vi "Translate Tile.vi"(0 "Tile in":T2 items=["Empty", "Portal", "Open", "Wall", ">", "<", ">-^", ">-v", "^-<", "v-<"], 1 "Direction in":T1) -> (2 "Direction out":T1, 3 "Tile out":T2 items=["Empty", "Portal", "Open", "Wall", ">", "<", ">-^", ">-v", "^-<", "v-<"])   [LabVIEW 2020, in "AoC 2022.lvlib"]
uses:
  AoC 2022.lvlib
  Map Tile.ctl
  Map Direction.ctl
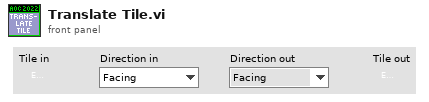
[diagram p1: front panel]
types:
  T1 = typedef "AoC 2022.lvlib/Map Direction.ctl" = enum16{"Facing", "Right", "Left", "Up", "Down"}
  T2 = typedef "AoC 2022.lvlib/Map Tile.ctl" = u16
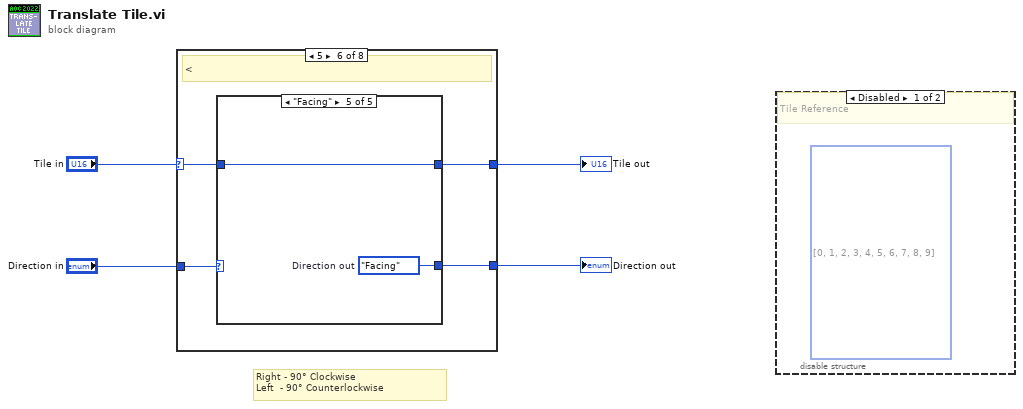
[diagram p0: block diagram]
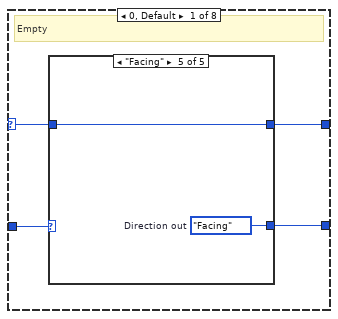
[diagram p2: hidden frame]
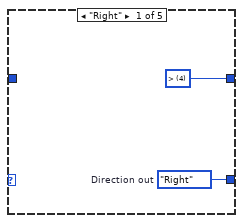
[diagram p3: hidden frame]
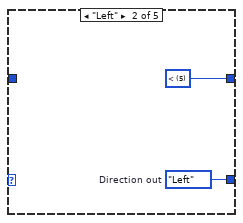
[diagram p4: hidden frame]
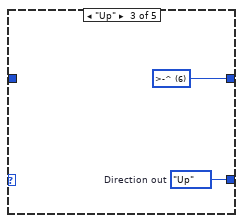
[diagram p5: hidden frame]
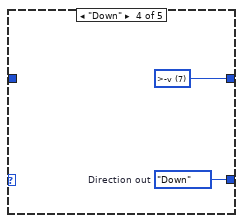
[diagram p6: hidden frame]
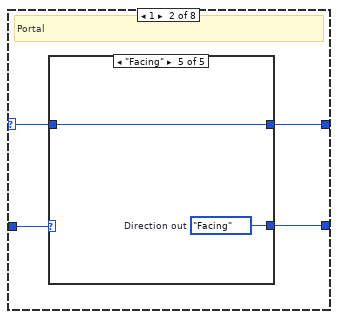
[diagram p7: hidden frame]
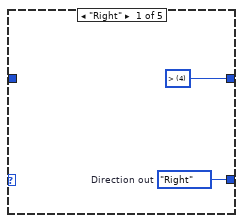
[diagram p8: hidden frame]
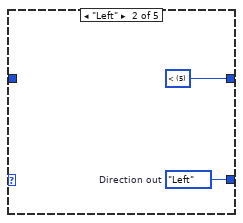
[diagram p9: hidden frame]
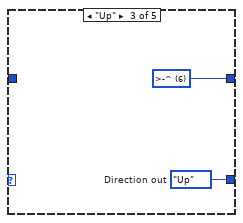
[diagram p10: hidden frame]
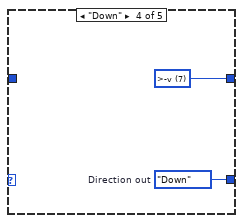
[diagram p11: hidden frame]
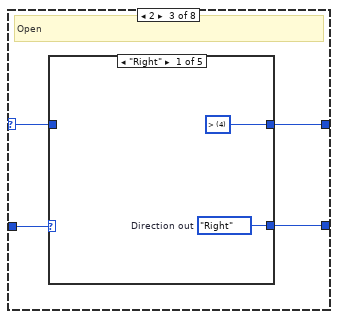
[diagram p12: hidden frame]
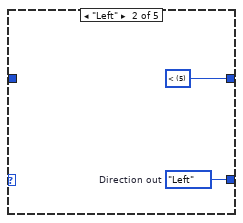
[diagram p13: hidden frame]
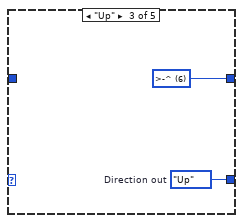
[diagram p14: hidden frame]
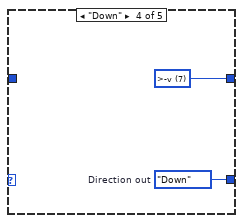
[diagram p15: hidden frame]
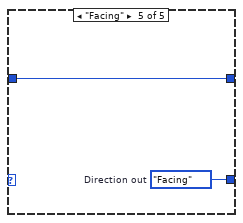
[diagram p16: hidden frame]
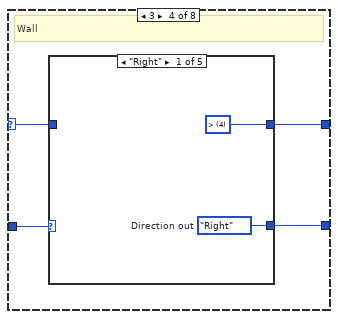
[diagram p17: hidden frame]
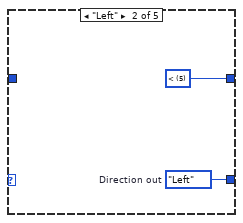
[diagram p18: hidden frame]
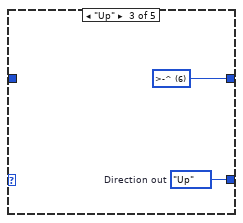
[diagram p19: hidden frame]
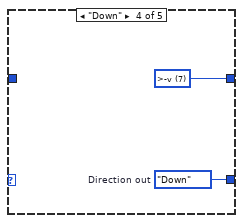
[diagram p20: hidden frame]
diagram:
  # "Right - 90° Clockwise\nLeft  - 90° Counterlockwise"
  n1 = case shown="5" "Tile in" {
    selector: "Tile in" -> [w5 w19 w33 w47 w61 w75 w89 w103]
    tunnel: [w8 w22 w36 w50 w64 w78 w92 w106] -> w3
    tunnel: "Direction in" -> [w7 w21 w35 w49 w63 w77 w91 w105]
    tunnel: [w6 w20 w34 w48 w62 w76 w90 w104] -> w1
    frame 0, Default {
      # "Empty"
      n2 = case shown="\"Facing\"" w7 {
        tunnel: [w10 w12 w14 w16 w17] -> w8
        tunnel: [w9 w11 w13 w15 w18] -> w6
        tunnel: w5 -> [_ _ _ _ w17]
        frame "Right" {
          w9 = Map_Direction."Right"  # Direction out
          w10 = T2 4 items=["Empty", "Portal", "Open", "Wall", ">", "<", ">-^", ">-v", "^-<", "v-<"] ("Tile")
        }
        frame "Left" {
          w11 = Map_Direction."Left"  # Direction out
          w12 = T2 5 items=["Empty", "Portal", "Open", "Wall", ">", "<", ">-^", ">-v", "^-<", "v-<"] ("Tile")
        }
        frame "Up" {
          w13 = Map_Direction."Up"  # Direction out
          w14 = T2 6 items=["Empty", "Portal", "Open", "Wall", ">", "<", ">-^", ">-v", "^-<", "v-<"] ("Tile")
        }
        frame "Down" {
          w15 = Map_Direction."Down"  # Direction out
          w16 = T2 7 items=["Empty", "Portal", "Open", "Wall", ">", "<", ">-^", ">-v", "^-<", "v-<"] ("Tile")
        }
        frame "Facing" {
          w18 = Map_Direction."Facing"  # Direction out
        }
      }
    }
    frame 1 {
      # "Portal"
      n3 = case shown="\"Facing\"" w21 {
        tunnel: [w24 w26 w28 w30 w31] -> w22
        tunnel: [w23 w25 w27 w29 w32] -> w20
        tunnel: w19 -> [_ _ _ _ w31]
        frame "Right" {
          w23 = Map_Direction."Right"  # Direction out
          w24 = T2 4 items=["Empty", "Portal", "Open", "Wall", ">", "<", ">-^", ">-v", "^-<", "v-<"] ("Tile")
        }
        frame "Left" {
          w25 = Map_Direction."Left"  # Direction out
          w26 = T2 5 items=["Empty", "Portal", "Open", "Wall", ">", "<", ">-^", ">-v", "^-<", "v-<"] ("Tile")
        }
        frame "Up" {
          w27 = Map_Direction."Up"  # Direction out
          w28 = T2 6 items=["Empty", "Portal", "Open", "Wall", ">", "<", ">-^", ">-v", "^-<", "v-<"] ("Tile")
        }
        frame "Down" {
          w29 = Map_Direction."Down"  # Direction out
          w30 = T2 7 items=["Empty", "Portal", "Open", "Wall", ">", "<", ">-^", ">-v", "^-<", "v-<"] ("Tile")
        }
        frame "Facing" {
          w32 = Map_Direction."Facing"  # Direction out
        }
      }
    }
    frame 2 {
      # "Open"
      n4 = case shown="\"Right\"" w35 {
        tunnel: [w38 w40 w42 w44 w45] -> w36
        tunnel: [w37 w39 w41 w43 w46] -> w34
        tunnel: w33 -> [_ _ _ _ w45]
        frame "Right" {
          w37 = Map_Direction."Right"  # Direction out
          w38 = T2 4 items=["Empty", "Portal", "Open", "Wall", ">", "<", ">-^", ">-v", "^-<", "v-<"] ("Tile")
        }
        frame "Left" {
          w39 = Map_Direction."Left"  # Direction out
          w40 = T2 5 items=["Empty", "Portal", "Open", "Wall", ">", "<", ">-^", ">-v", "^-<", "v-<"] ("Tile")
        }
        frame "Up" {
          w41 = Map_Direction."Up"  # Direction out
          w42 = T2 6 items=["Empty", "Portal", "Open", "Wall", ">", "<", ">-^", ">-v", "^-<", "v-<"] ("Tile")
        }
        frame "Down" {
          w43 = Map_Direction."Down"  # Direction out
          w44 = T2 7 items=["Empty", "Portal", "Open", "Wall", ">", "<", ">-^", ">-v", "^-<", "v-<"] ("Tile")
        }
        frame "Facing" {
          w46 = Map_Direction."Facing"  # Direction out
        }
      }
    }
    frame 3 {
      # "Wall"
      n5 = case shown="\"Right\"" w49 {
        tunnel: [w52 w54 w56 w58 w59] -> w50
        tunnel: [w51 w53 w55 w57 w60] -> w48
        tunnel: w47 -> [_ _ _ _ w59]
        frame "Right" {
          w51 = Map_Direction."Right"  # Direction out
          w52 = T2 4 items=["Empty", "Portal", "Open", "Wall", ">", "<", ">-^", ">-v", "^-<", "v-<"] ("Tile")
        }
        frame "Left" {
          w53 = Map_Direction."Left"  # Direction out
          w54 = T2 5 items=["Empty", "Portal", "Open", "Wall", ">", "<", ">-^", ">-v", "^-<", "v-<"] ("Tile")
        }
        frame "Up" {
          w55 = Map_Direction."Up"  # Direction out
          w56 = T2 6 items=["Empty", "Portal", "Open", "Wall", ">", "<", ">-^", ">-v", "^-<", "v-<"] ("Tile")
        }
        frame "Down" {
          w57 = Map_Direction."Down"  # Direction out
          w58 = T2 7 items=["Empty", "Portal", "Open", "Wall", ">", "<", ">-^", ">-v", "^-<", "v-<"] ("Tile")
        }
        frame "Facing" {
          w60 = Map_Direction."Facing"  # Direction out
        }
      }
    }
    frame 4 {
      # ">"
      n6 = case shown="\"Left\"" w63 {
        tunnel: [w66 w68 w70 w72 w73] -> w64
        tunnel: [w65 w67 w69 w71 w74] -> w62
        tunnel: w61 -> [_ _ _ _ w73]
        frame "Right" {
          w65 = Map_Direction."Down"  # Direction out
          w66 = T2 7 items=["Empty", "Portal", "Open", "Wall", ">", "<", ">-^", ">-v", "^-<", "v-<"] ("Tile")
        }
        frame "Left" {
          w67 = Map_Direction."Up"  # Direction out
          w68 = T2 6 items=["Empty", "Portal", "Open", "Wall", ">", "<", ">-^", ">-v", "^-<", "v-<"] ("Tile")
        }
        frame "Up" {
          w69 = Map_Direction."Up"  # Direction out
          w70 = T2 6 items=["Empty", "Portal", "Open", "Wall", ">", "<", ">-^", ">-v", "^-<", "v-<"] ("Tile")
        }
        frame "Down" {
          w71 = Map_Direction."Down"  # Direction out
          w72 = T2 7 items=["Empty", "Portal", "Open", "Wall", ">", "<", ">-^", ">-v", "^-<", "v-<"] ("Tile")
        }
        frame "Facing" {
          w74 = Map_Direction."Facing"  # Direction out
        }
      }
    }
    frame 5 {
      # "<"
      n7 = case shown="\"Facing\"" w77 {
        tunnel: [w80 w82 w84 w86 w87] -> w78
        tunnel: [w79 w81 w83 w85 w88] -> w76
        tunnel: w75 -> [_ _ _ _ w87]
        frame "Right" {
          w79 = Map_Direction."Up"  # Direction out
          w80 = T2 8 items=["Empty", "Portal", "Open", "Wall", ">", "<", ">-^", ">-v", "^-<", "v-<"] ("Tile")
        }
        frame "Left" {
          w81 = Map_Direction."Down"  # Direction out
          w82 = T2 9 items=["Empty", "Portal", "Open", "Wall", ">", "<", ">-^", ">-v", "^-<", "v-<"] ("Tile")
        }
        frame "Up" {
          w83 = Map_Direction."Up"  # Direction out
          w84 = T2 8 items=["Empty", "Portal", "Open", "Wall", ">", "<", ">-^", ">-v", "^-<", "v-<"] ("Tile")
        }
        frame "Down" {
          w85 = Map_Direction."Down"  # Direction out
          w86 = T2 7 items=["Empty", "Portal", "Open", "Wall", ">", "<", ">-^", ">-v", "^-<", "v-<"] ("Tile")
        }
        frame "Facing" {
          w88 = Map_Direction."Facing"  # Direction out
        }
      }
    }
    frame 6, 8 {
      # "^"
      n8 = case shown="\"Facing\"" w91 {
        tunnel: [w94 w96 w98 w100 w101] -> w92
        tunnel: [w93 w95 w97 w99 w102] -> w90
        tunnel: w89 -> [_ _ _ _ w101]
        frame "Right" {
          w93 = Map_Direction."Right"  # Direction out
          w94 = T2 4 items=["Empty", "Portal", "Open", "Wall", ">", "<", ">-^", ">-v", "^-<", "v-<"] ("Tile")
        }
        frame "Left" {
          w95 = Map_Direction."Left"  # Direction out
          w96 = T2 5 items=["Empty", "Portal", "Open", "Wall", ">", "<", ">-^", ">-v", "^-<", "v-<"] ("Tile")
        }
        frame "Up" {
          w97 = Map_Direction."Up"  # Direction out
          w98 = T2 8 items=["Empty", "Portal", "Open", "Wall", ">", "<", ">-^", ">-v", "^-<", "v-<"] ("Tile")
        }
        frame "Down" {
          w99 = Map_Direction."Down"  # Direction out
          w100 = T2 7 items=["Empty", "Portal", "Open", "Wall", ">", "<", ">-^", ">-v", "^-<", "v-<"] ("Tile")
        }
        frame "Facing" {
          w102 = Map_Direction."Facing"  # Direction out
        }
      }
    }
    frame 7, 9 {
      # "v"
      n9 = case shown="\"Right\"" w105 {
        tunnel: [w108 w110 w112 w114 w115] -> w106
        tunnel: [w107 w109 w111 w113 w116] -> w104
        tunnel: w103 -> [_ _ _ _ w115]
        frame "Right" {
          w107 = Map_Direction."Left"  # Direction out
          w108 = T2 5 items=["Empty", "Portal", "Open", "Wall", ">", "<", ">-^", ">-v", "^-<", "v-<"] ("Tile")
        }
        frame "Left" {
          w109 = Map_Direction."Right"  # Direction out
          w110 = T2 4 items=["Empty", "Portal", "Open", "Wall", ">", "<", ">-^", ">-v", "^-<", "v-<"] ("Tile")
        }
        frame "Up" {
          w111 = Map_Direction."Up"  # Direction out
          w112 = T2 8 items=["Empty", "Portal", "Open", "Wall", ">", "<", ">-^", ">-v", "^-<", "v-<"] ("Tile")
        }
        frame "Down" {
          w113 = Map_Direction."Down"  # Direction out
          w114 = T2 7 items=["Empty", "Portal", "Open", "Wall", ">", "<", ">-^", ">-v", "^-<", "v-<"] ("Tile")
        }
        frame "Facing" {
          w116 = Map_Direction."Facing"  # Direction out
        }
      }
    }
  }
  "Tile out" <- w3
  "Direction out" <- w1
  n10 = disable-structure shown="Disabled" {
    frame Disabled {
      (unwired) T2[] [0, 1, 2, 3, 4, 5, 6, 7, 8, 9] items=["Empty", "Portal", "Open", "Wall", ">", "<", ">-^", ">-v", "^-<", "v-<"]
      # "Tile Reference"
    }
    frame Enabled {
    }
  }
